vi "Diagnostic Measurment.vi"(8 "error in (no error)":errorcluster, 11 "MSX-E3711 in":refnum<class "MSX-E3711.lvclass">) -> (0 "error out":errorcluster, 3 "MSX-E3711 out":refnum<class "MSX-E3711.lvclass">)   [LabVIEW 2014, in "MSX-E3711.lvlib" / "MSX-E3711.lvclass"]
uses:
  MSX-E3711.lvclass
  MSX-E3711.lvclass/MSX-E3711.ctl
  DriverMasterSync/build/DriverMasterSync.lvlibp/Modules/HAL/DriverMasterSync/DriverMasterSyncClass/DriverMasterSync.lvclass
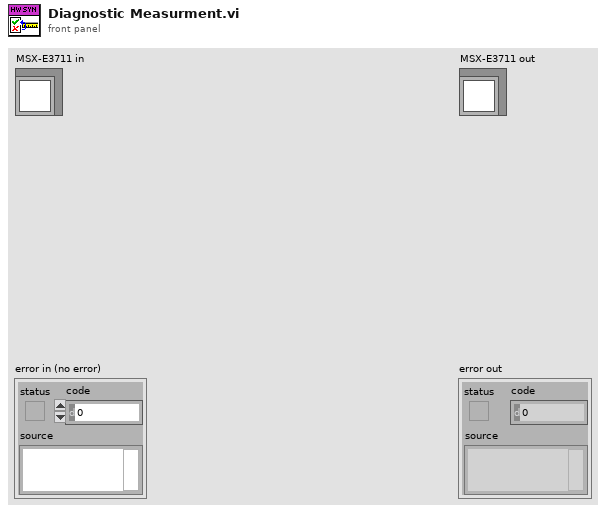
[diagram p1: front panel]
types:
  T1 = typedef "DriverMasterSync.lvlibp/HAL Config Data.ctl" = cluster{"HWSync Index":u32, "Driver Name":string, "Channel Mask":u64}
  T2 = typedef "DriverMasterSync.lvlibp/WINFAS 2 Data Queue.lvlib/Acquisition Data 1 Sample Cluster.ctl" = cluster{"TDX":sgl[], "Encoder":sgl}
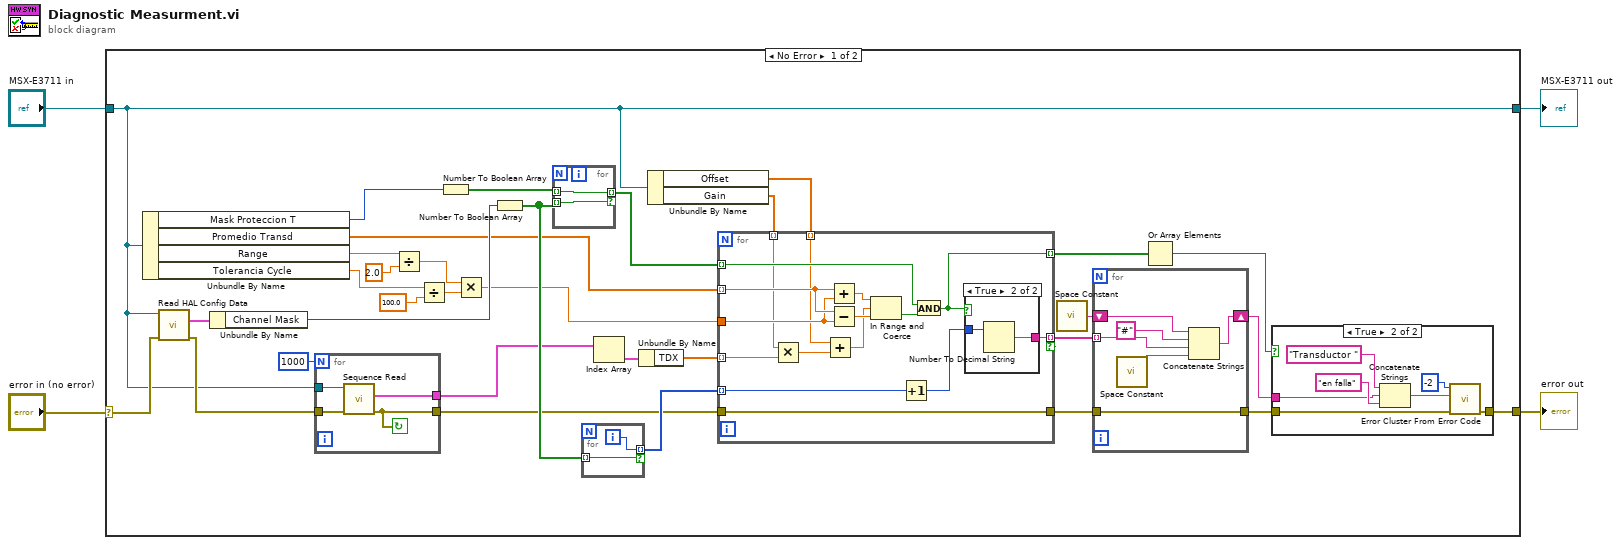
[diagram p0: block diagram]
diagram:
  n1 = case shown="No Error" "error in (no error)" {
    selector: "error in (no error)" -> [w11 w79]
    tunnel: [w10 w79] -> w3
    tunnel: [w5 w78] -> w1
    tunnel: "MSX-E3711 in" -> [w5 w78]
    frame No Error {
      n2 = Unbundle By Name(w5) -> ("Mask Proteccion T"=w36:u64, "Promedio Transd"=w21:sgl[], "Range"=w16:sgl, "Tolerancia Cycle"=w15:sgl)
      n3 = call "Read HAL Config Data.vi"("error in (no error)"=w11, "DriverMasterSync in"=w5) -> ("error out"=w6:errorcluster, "HAL Config Data"=w12:T1)  [unwired: 7 in, 1 out]
      n4 = Unbundle By Name(w12) -> ("Channel Mask"=w27:u64)
      n5 = for {
        N: 1000 -> [_]
        tunnel: [w39] -> w8
        tunnel: [w40] -> w7
        tunnel: w6 -> [w41]
        tunnel: w5 -> [w38]
        stop <- w40 continue-if-true
        n6 = call-dynamic "Sequence Read.vi"("error in (no error)"=w41, "MSX-E3711 in"=w38) -> ("error out"=w40:errorcluster, "Acquisition Data"=w39:T2[])  [unwired: 6 in, 2 out]
      }
      n7 = Divide(x=w16, y=sgl 2.0) -> (x/y=w18:sgl)
      n8 = Divide(x=w15, y=sgl 100.0) -> (x/y=w37:sgl)
      n9 = Number To Boolean Array(number=w36) -> (Boolean array=w24:bool[])
      n10 = Multiply(x=w18, y=w37) -> (x*y=w20:sgl)
      n11 = Number To Boolean Array(number=w27) -> (Boolean array=w23:bool[])
      n12 = for {
        tunnel: w24 -> [w45] mode=indexing
        tunnel: [w45] -> w28 mode=indexing if=w44
        tunnel: w23 -> [w44] mode=indexing
      }
      n13 = for {
        tunnel: w23 -> [w42] mode=indexing
        tunnel: [w43] -> w22 mode=indexing if=w42
        i -> [w43]
      }
      n14 = Index Array(array=w8) -> (element=w26:T2)  [unwired: 1 in]
      n15 = Unbundle By Name(w26) -> ("TDX"=w25:sgl[])
      n16 = Unbundle By Name(w5) -> ("Offset"=w13:sgl[], "Gain"=w14:sgl[])
      n17 = for {
        tunnel: w7 -> [w75]
        tunnel: w28 -> [w72] mode=indexing
        tunnel: [w75] -> w32
        tunnel: [w71] -> w35 mode=indexing
        tunnel: [w73] -> w30 mode=indexing if=w71
        tunnel: w25 -> [w62] mode=indexing
        tunnel: w22 -> [w69] mode=indexing
        tunnel: w21 -> [w68] mode=indexing
        tunnel: w20 -> [w67]
        tunnel: w14 -> [w61] mode=indexing
        tunnel: w13 -> [w60] mode=indexing
        n18 = Multiply(x=w61, y=w62) -> (x*y=w64:sgl)
        n19 = Add(x=w60, y=w64) -> (x+y=w63:sgl)
        n20 = Add(x=w68, y=w67) -> (x+y=w66:sgl)
        n21 = Subtract(x=w68, y=w67) -> (x-y=w65:sgl)
        n22 = In Range and Coerce(upper limit=w66, x=w63, lower limit=w65) -> (In Range?=w74:bool)  [unwired: 1 out]
        n23 = Increment(x=w69) -> (x+1=w70:i32)
        n24 = And(x=w72, y=w74) -> (x .and. y?=w71:bool)
        n25 = case shown="True" w71 {
          tunnel: w70 -> [_ w77]
          tunnel: [_ w76] -> w73
          frame False {
          }
          frame True {
            n26 = Number To Decimal String(number=w77) -> (decimal integer string=w76:string)  [unwired: 1 in]
          }
        }
      }
      n27 = call <vilib>:"Space Constant.vi"() -> ("String"=w31:string)
      n28 = for {
        tunnel: [w51] -> w33
        tunnel: w32 -> [w51]
        shift-right: [w50] -> w29
        shift-left: w31 -> [w49]
        tunnel: w30 -> [w47] mode=indexing
        n29 = call <vilib>:"Space Constant.vi"() -> ("String"=w46:string)
        n30 = Concatenate Strings(w49, "#" ("string"), w47, w46) -> (w50:string)
      }
      n31 = Or Array Elements(Boolean array=w35) -> (logical OR=w34:bool)
      n32 = case shown="True" w34 {
        tunnel: w33 -> [w52 w55]
        tunnel: [w52 w54] -> w10
        tunnel: w29 -> [_ w53]
        frame False {
        }
        frame True {
          n33 = Concatenate Strings("Transductor ", w53, "en falla" ("string")) -> (w56:string)
          n34 = call <vilib>:"Error Cluster From Error Code.vi"("error in (no error)"=w55, "error message (\"\")"=w56, "error code (0)"=-2) -> ("error out"=w54:errorcluster)  [unwired: 6 in]
        }
      }
    }
    frame Error {
    }
  }
  "error out" <- w3
  "MSX-E3711 out" <- w1
